vi "Progetto C - analisi dimensionale.vi"() -> ()   [LabVIEW 2020]
panel:
  in  "In/Out_Pannel":enum32{"Input", "Output"}(tab)
  in  "STOP":bool
  in  "Saving File Path":path
  in  "Sensors_Distance [mm]":dbl
  in  "Max_Time [s]":dbl
  out "Data":string[][](array[string])
  out "E[Speed]":dbl format="%0.2f"
  out "Var[Speed]":dbl format="%0.5f"
  out "E[Length]":dbl format="%0.2f"
  out "Var[Length]":dbl format="%0.2f"
  out "Histogram_Speed":T1(graph)
  out "Histogram_Length":T1(graph)
  out "Success %":dbl
  out "S2":bool
  out "S1":bool
  out "Alarm":bool
  out "Length [mm]":dbl
  out "Speed [mm/s]":dbl
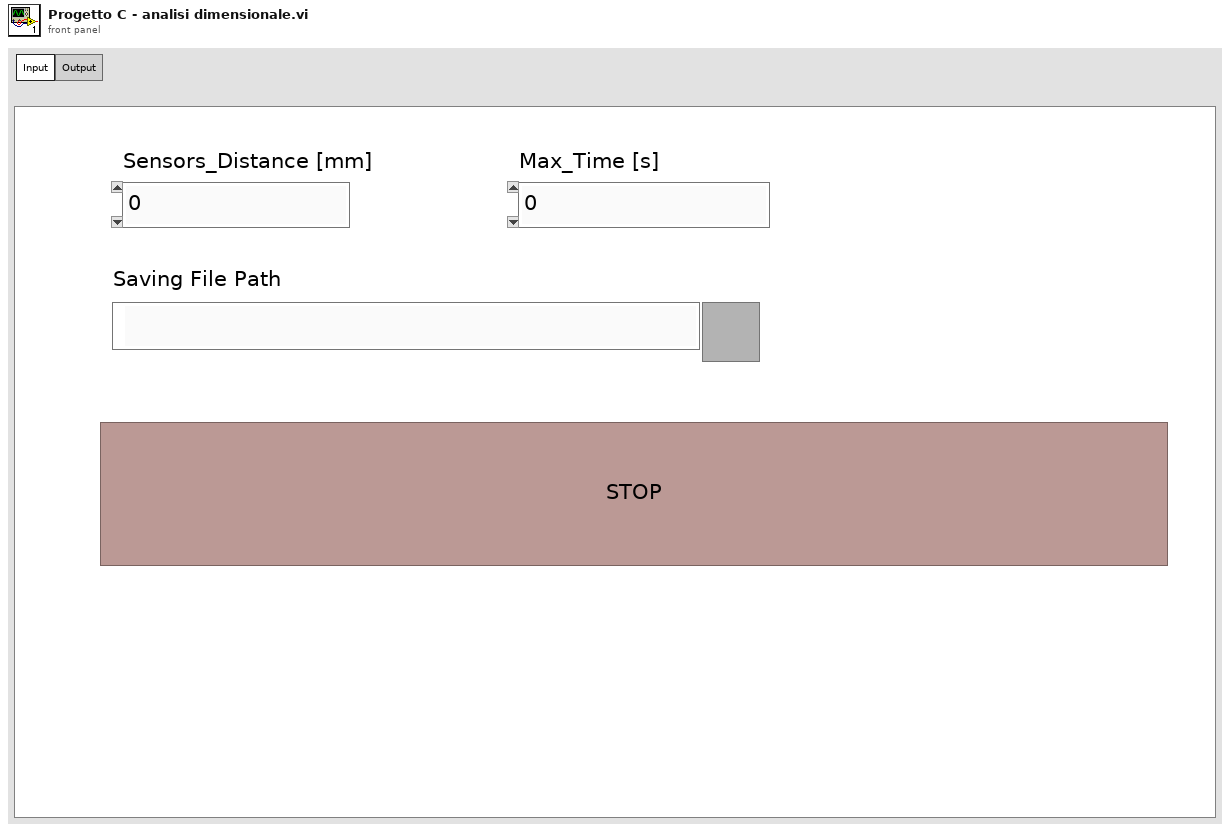
[diagram p1: front panel]
types:
  T1 = cluster{"X Values":dbl[], "Histogram: h(x)":i32[]}
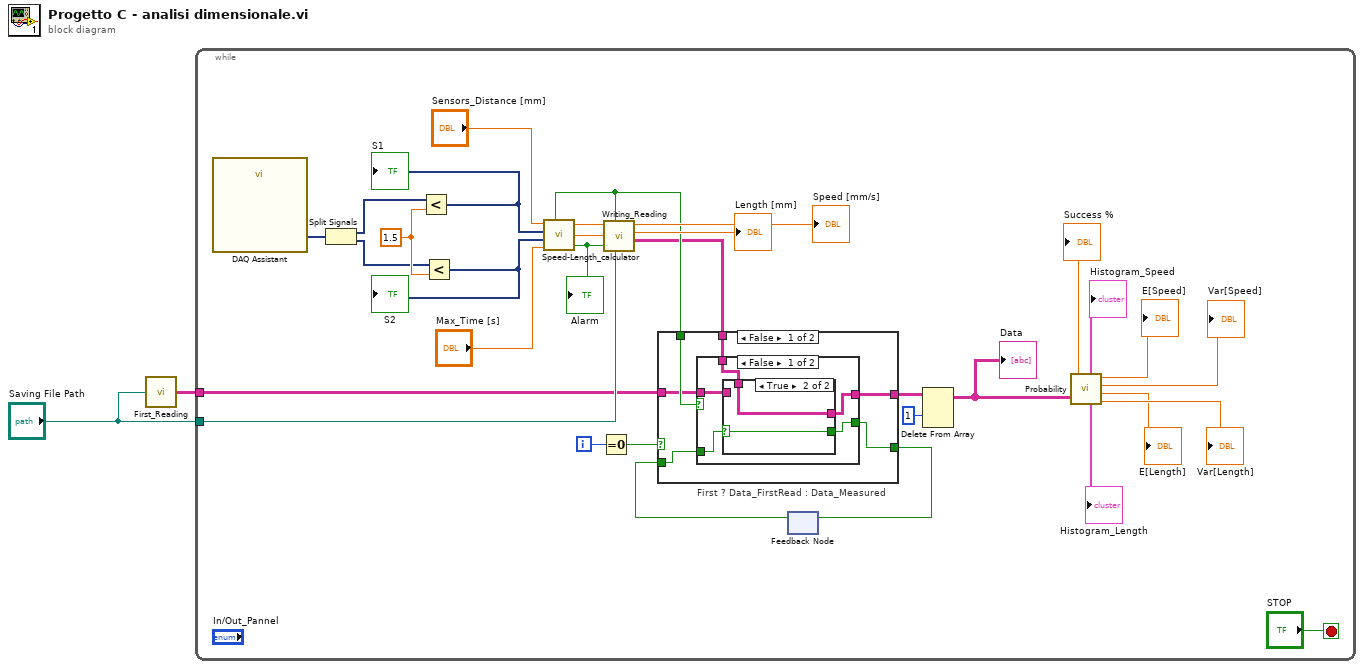
[diagram p0: block diagram]
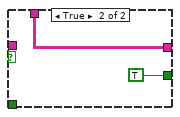
[diagram p3: hidden frame]
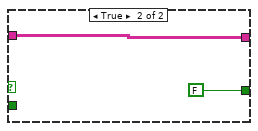
[diagram p4: hidden frame]
diagram:
  n1 = call "First_Reading.vi"("Saving File Path"="Saving File Path") -> ("Data"=w2:string[][])
  n2 = while {
    tunnel: "Saving File Path" -> [w28]
    tunnel: w2 -> [w26]
    i -> [w27]
    stop <- "STOP" stop-if-true
    w11 = 1.5 ("y")
    n3 = call "DAQ Assistant"() -> ("data"=w10:dynamicdata)  [unwired: 16 in, 3 out]
    n4 = Split Signals(w10) -> (w8:dynamicdata, w7:dynamicdata)  [unwired: 2 in]
    n5 = Less?(x=w8, y=w11) -> (x < y?=w9:dynamicdata)
    "S1" <- w9
    n6 = Less?(x=w7, y=w11) -> (x < y?=w6:dynamicdata)
    "S2" <- w6
    n7 = call "Speed-Length_calculator.vi"("Sensors_Distance [mm]"="Sensors_Distance [mm]", "TriggerS1"=w9, "TriggerS2"=w6, "Max_Time [s]"="Max_Time [s]") -> ("Flag_EndMeasure"=w24:bool, "Speed [mm/s]"=w33:dbl, "Length [mm]"=w32:dbl, "Alarm"=w29:bool)
    "Alarm" <- w29
    n8 = Equal To 0?(x=w27) -> (x = 0?=w25:bool)
    n9 = call "Writing_Reading.vi"("Saving File Path"=w28, "Enable"=w24, "Alarm_IN"=w29, "Length_IN"=w32, "Speed_IN"=w33) -> ("data"=w23:string[][], "Length_OUT"=→"Length [mm]":dbl, "Speed_OUT"=→"Speed [mm/s]":dbl)  [unwired: 1 in, 1 out]
    n10 = feedback #1() -> (w21:bool)  [unwired: 1 in]
    n11 = case "First ? Data_FirstRead : Data_Measured" shown="False" w25 {
      tunnel: w26 -> [w36 w53]
      tunnel: [w38 w53] -> w20
      tunnel: w24 -> [w40 _]
      tunnel: w23 -> [w39 _]
      tunnel: [w35 FALSE] -> w22
      tunnel: w21 -> [w37 _]
      frame False {
        n12 = case shown="False" w40 {
          tunnel: w39 -> [w41 w51]
          tunnel: [w43 w51] -> w38
          tunnel: w37 -> [w45 _]
          tunnel: w36 -> [w44 _]
          tunnel: [w42 TRUE] -> w35
          frame False {
            n13 = case shown="True" w45 {
              selector: w45 -> [w46 w48]
              tunnel: w44 -> [w47 _]
              tunnel: [w47 w49] -> w43
              tunnel: [w46 w48] -> w42
              tunnel: w41 -> [_ w49]
              frame False {
              }
              frame True {
              }
            }
          }
          frame True {
          }
        }
      }
      frame True {
      }
    }
    n14 = feedback-in #1(w22) -> ()
    n15 = Delete From Array(array=w20, index (row)=1) -> (array with subset deleted=w18:string[][])  [unwired: 2 in, 1 out]
    "Data" <- w18
    n16 = call "Probability.vi"("Data"=w18) -> ("Success %"=→"Success %":dbl, "Histogram_Speed"=→"Histogram_Speed":T1, "Histogram_Length"=→"Histogram_Length":T1, "E[Speed]"=→"E[Speed]":dbl, "Var[Speed]"=→"Var[Speed]":dbl, "E[Length]"=→"E[Length]":dbl, "Var[Length]"=→"Var[Length]":dbl)
  }
